vi "PXI_Host_U16_Write_NewMethod_Benchmark.vi"() -> ()   [LabVIEW 2018]
uses:
  cRIO RT/FPGA Bitfile Register Operations/Scalar IO Operations/Write Methods/Write Data Register/Instances/Write U16.vi
  cRIO RT/FPGA Bitfile Register Operations/Scalar IO Operations/Utilities/Find Register Offset.vi
  cRIO RT/FPGA Bitfile Register Operations/Scalar IO Operations/SubVIs/Check Register Data Store.vi
  cRIO RT/FPGA Bitfile Register Operations/Scalar IO Operations/Error Handling/Error 6001.vi
  cRIO RT/FPGA Bitfile Register Operations/Scalar IO Operations/Error Handling/Error 6000.vi
  cRIO RT/FPGA Bitfile Register Operations/Scalar IO Operations/Error Handling/Error 6002.vi
  cRIO RT/FPGA Bitfile Register Operations/Scalar IO Operations/Error Handling/Error 6006.vi
  <vilib>/FPGAPlugInAG/Dynamic/niLvFpga_Close_Dynamic.vi
  <vilib>/rvi/interface/nirviCloseFPGA/nirviCloseFPGA.xnode
  cRIO RT/FPGA Bitfile Register Operations/Scalar IO Operations/FPGA Register IO.lvlib
panel:
  out "error out":errorcluster
  out "Execution time (s)":dbl
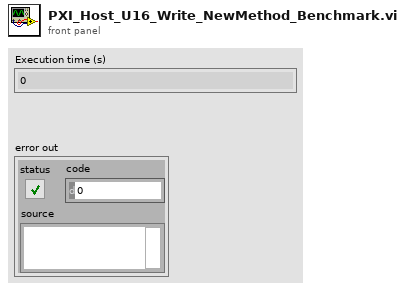
[diagram p1: front panel]
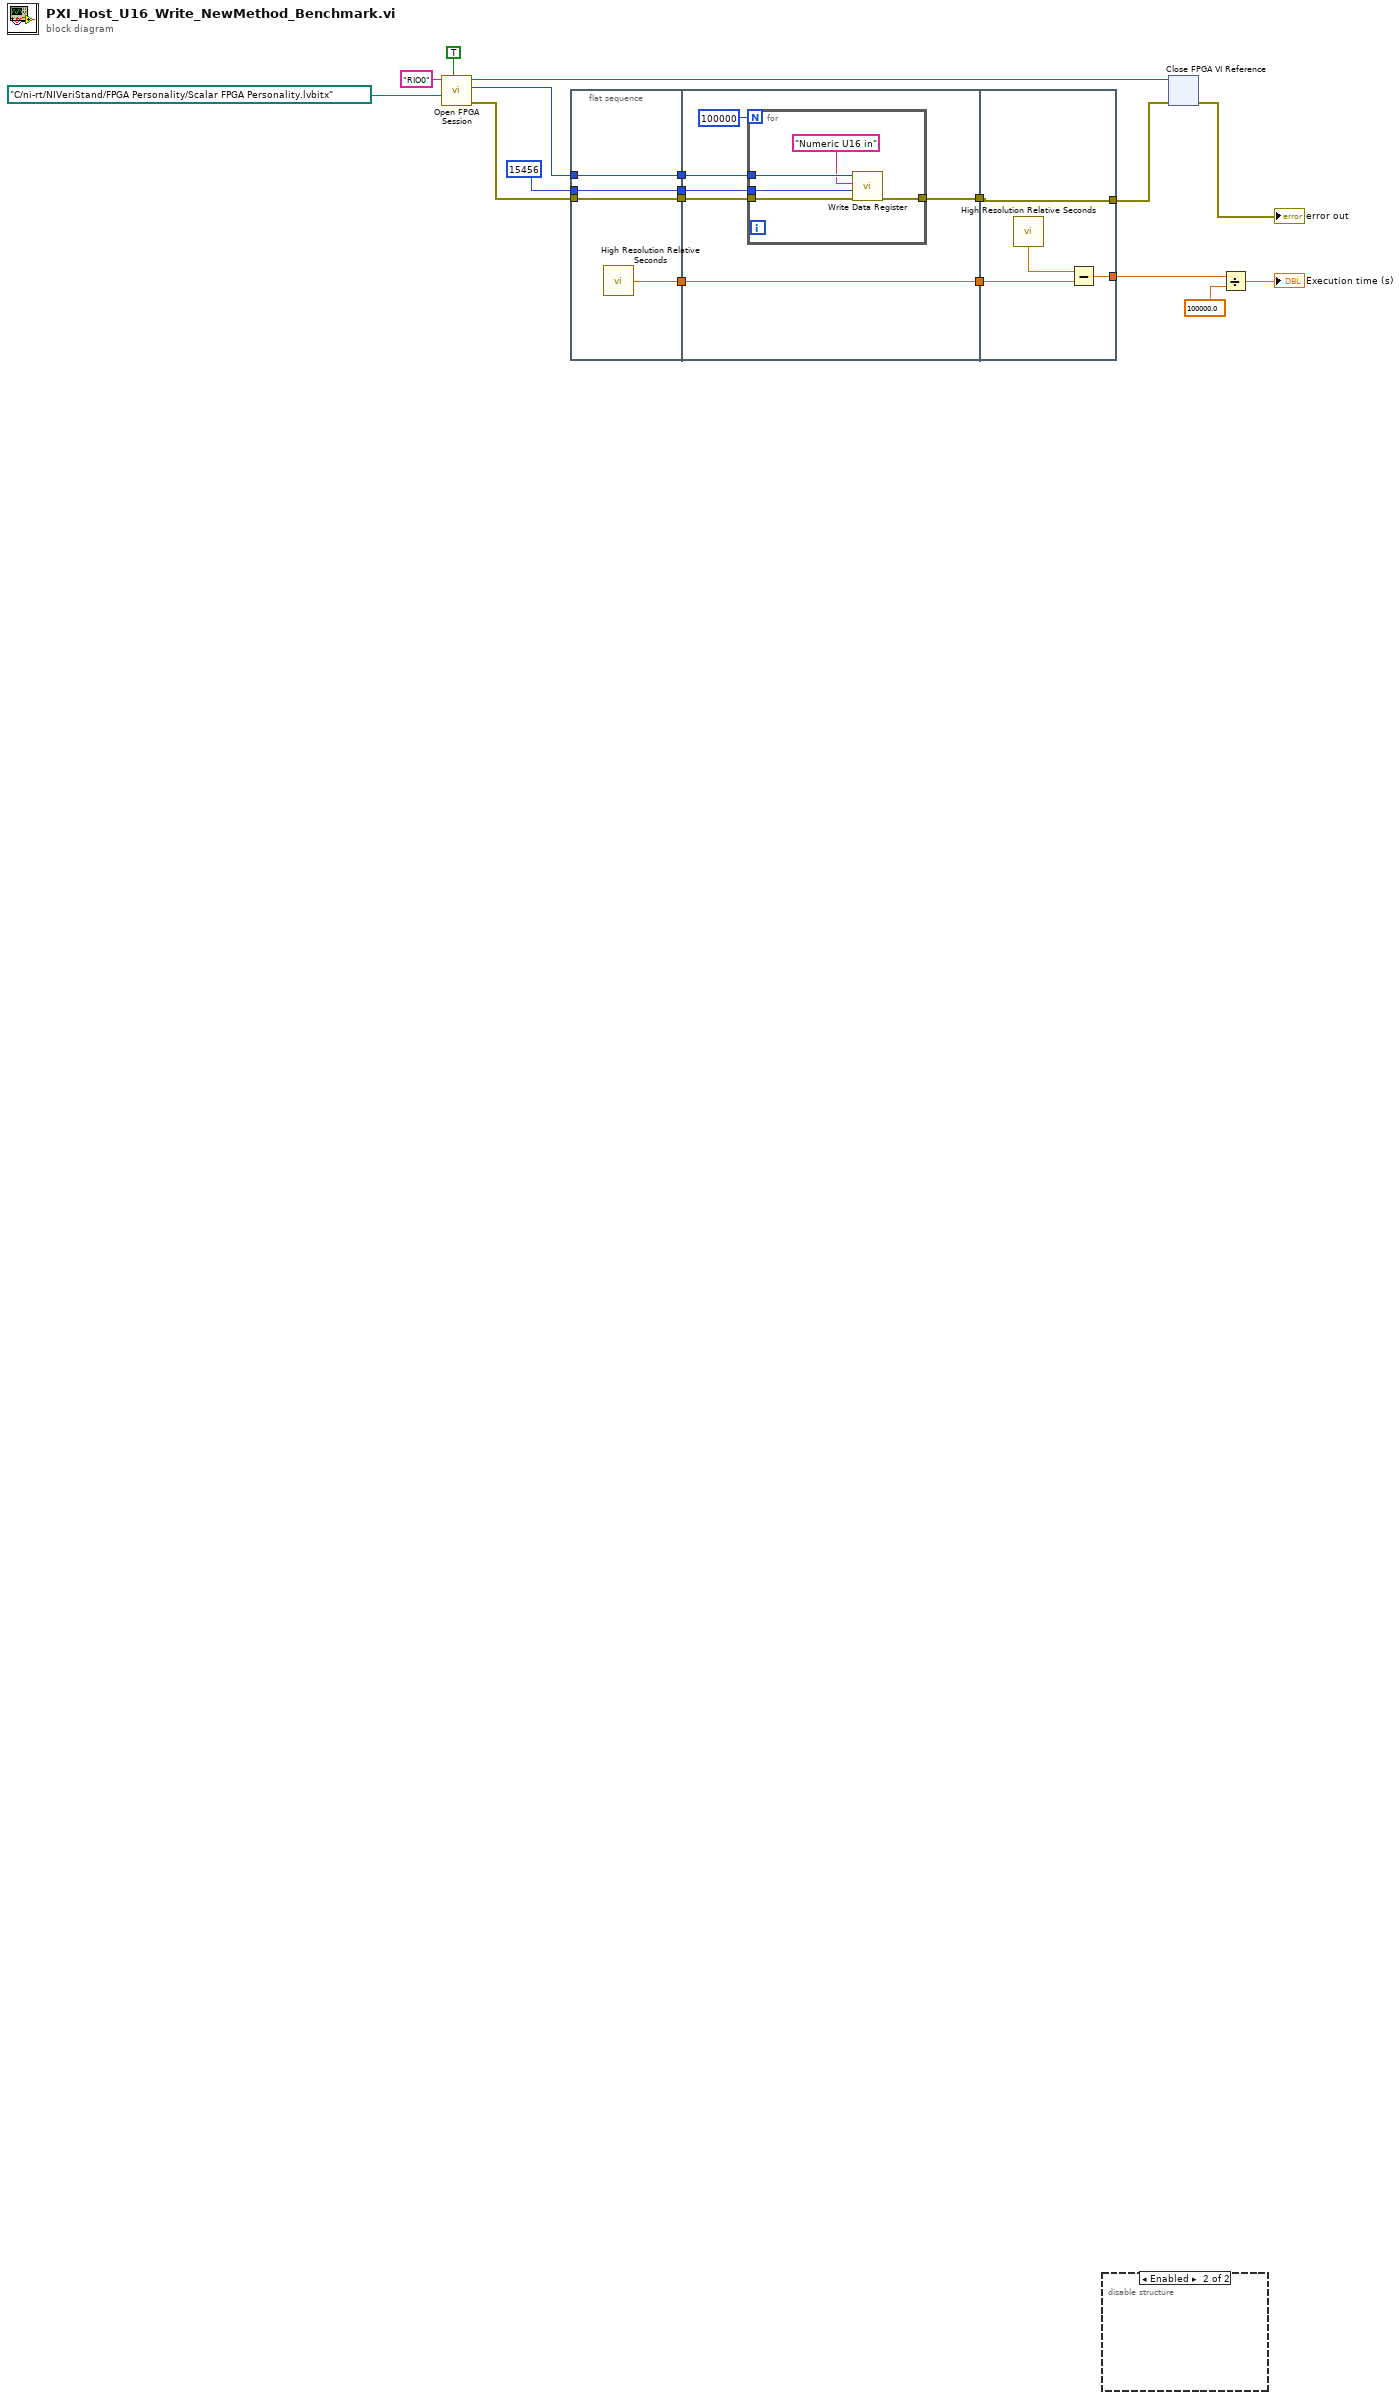
[diagram p0: block diagram]
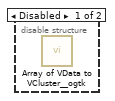
[diagram p2: hidden frame]
diagram:
  n1 = call "Open FPGA Session.vi"("run when loaded (T)"=TRUE, "bitfile path"=path "C:/ni-rt/NIVeriStand/FPGA Personality/Scalar FPGA Personality.lvbitx", "device address"="RIO0") -> ("error out"=w11:errorcluster, "session out"=w15:u32, "bitfile reference out"=w10:refnum<k20>)  [unwired: 6 in]
  n2 = flat-sequence {
    tunnel: [w22] -> w6
    tunnel: w15 -> [w21]
    tunnel: [w21] -> w5
    tunnel: w11 -> [w20]
    tunnel: [w20] -> w7
    tunnel: [w19] -> w2
    tunnel: u16 15456 ("value in") -> [w19]
    tunnel: [w27] -> w4
    tunnel: w6 -> [w27]
    tunnel: w5 -> [w26]
    tunnel: w7 -> [w25]
    tunnel: [w24] -> w3
    tunnel: w2 -> [w23]
    tunnel: w4 -> [w36]
    tunnel: [w35] -> w18
    tunnel: w3 -> [w34]
    tunnel: [w34] -> w9
    frame #0 {
      n3 = call <vilib>:"High Resolution Relative Seconds.vi"() -> ("relative seconds"=w22:dbl)
    }
    frame #1 {
      n4 = for {
        N: 100000 -> [_]
        tunnel: w26 -> [w31]
        tunnel: w25 -> [w33]
        tunnel: [w32] -> w24
        tunnel: w23 -> [w29]
        n5 = call-poly "Write Data Register.vi"("error in"=w33, "value in"=w29, "register name"="Numeric U16 in", "session in"=w31) -> ("error out"=w32:errorcluster)  [unwired: 6 in, 1 out]
      }
    }
    frame #2 {
      n6 = call <vilib>:"High Resolution Relative Seconds.vi"() -> ("relative seconds"=w37:dbl)
      n7 = Subtract(x=w37, y=w36) -> (x-y=w35:dbl)
    }
  }
  n8 = disable-structure shown="Enabled" {
    frame Disabled {
      n9 = call <userlib>:"Array of VData to VCluster__ogtk.vi"() -> ()  [unwired: 10 in, 2 out]
    }
    frame Enabled {
    }
  }
  n10 = xnode "Close FPGA VI Reference"("FPGA VI Reference In"=w10, "error in"=w9) -> ("error out"=→"error out":errorcluster)
  n11 = Divide(x=w18, y=100000.0) -> (x/y=→"Execution time (s)":dbl)
